vi "test.Cluster.vi"(8 "error in":errorcluster, 10 "Data":variant, 11 "Command":string) -> (0 "error out":errorcluster, 3 "Return Data":variant)   [LabVIEW 2014]
uses:
  Private/Class/class.GLue.lvclass
  Private/Class/meth.Constructor.vi
  Private/Class/meth.Destructor.vi
  GLue.lvlib
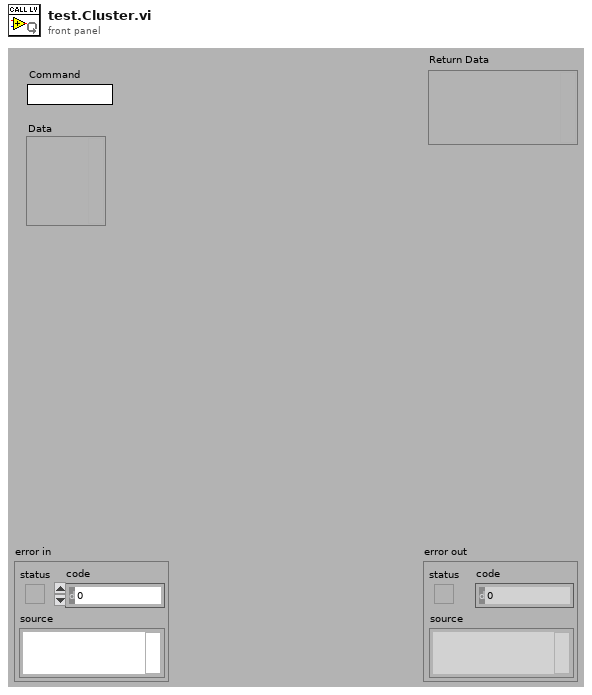
[diagram p1: front panel]
types:
  T1 = cluster{"bool":bool, "number":i32, "string":string, "ref":refnum<vi>}
  T2 = cluster{"ref":refnum<vi>, "df":string[][], "asd":cluster{"ref":refnum<vi>, "df":string[][]}[]}
  T3 = cluster{"arr":cluster{"ref":refnum<vi>, "df":string[][], "asd":cluster{"ref":refnum<vi>, "df":string[][]}[]}[]}
  T4 = cluster{"a":cluster{"bool":bool, "number":i32, "string":string}, "b":cluster{"bool":bool, "number":i32, "string":string, "c":cluster{"bool":bool, "number":i32, "string":string}}}
  T5 = cluster{"a":cluster{"bool":bool, "number":i32, "string":string}, "data":variant}
  T6 = cluster{"a":cluster{"numbers":i32[], "bools":bool[], "strings":string[]}, "b":cluster{"numbers":i32[], "bools":bool[], "strings":string[], "c":cluster{"numbers":i32[], "bools":bool[], "strings":string[]}}}
  T7 = cluster{"bool":bool, "number":i32, "string":string}
  T8 = cluster{"numbers":i32[], "bools":bool[], "strings":string[]}
  T9 = cluster{"numbers":i32[][], "bools":bool[][], "strings":string[][]}
  T10 = cluster{"ref":refnum<vi>, "df":string[][], "asd":cluster{"ref":refnum<vi>, "df":string[][]}[]}[]
  T11 = cluster{"a":refnum<vi>, "z":cluster{"array":string[][], "glue":refnum<class "class.GLue.lvclass">, "q":cluster{"a":refnum<vi>, "z":cluster{"array":string[][], "glue":refnum<class "class.GLue.lvclass">}[], "b":bool[], "c":refnum<queue>, "w":dbl[][], "d":cluster{"h":cluster{"i":picture, "j":variant, "g":path}, waveform(dbl)}}}[], "b":bool[], "c":refnum<queue>, "k 2":waveform(dbl), "d":cluster{"g":path, "h":cluster{"i":picture, "j":variant}}}
  T12 = cluster{"bool":bool, "number":i32, "string":string, "c":cluster{"bool":bool, "number":i32, "string":string}}
  T13 = cluster{"clus2":cluster{"clus1":cluster{bool, i32, "string":string}, string}, i32, "string":string}
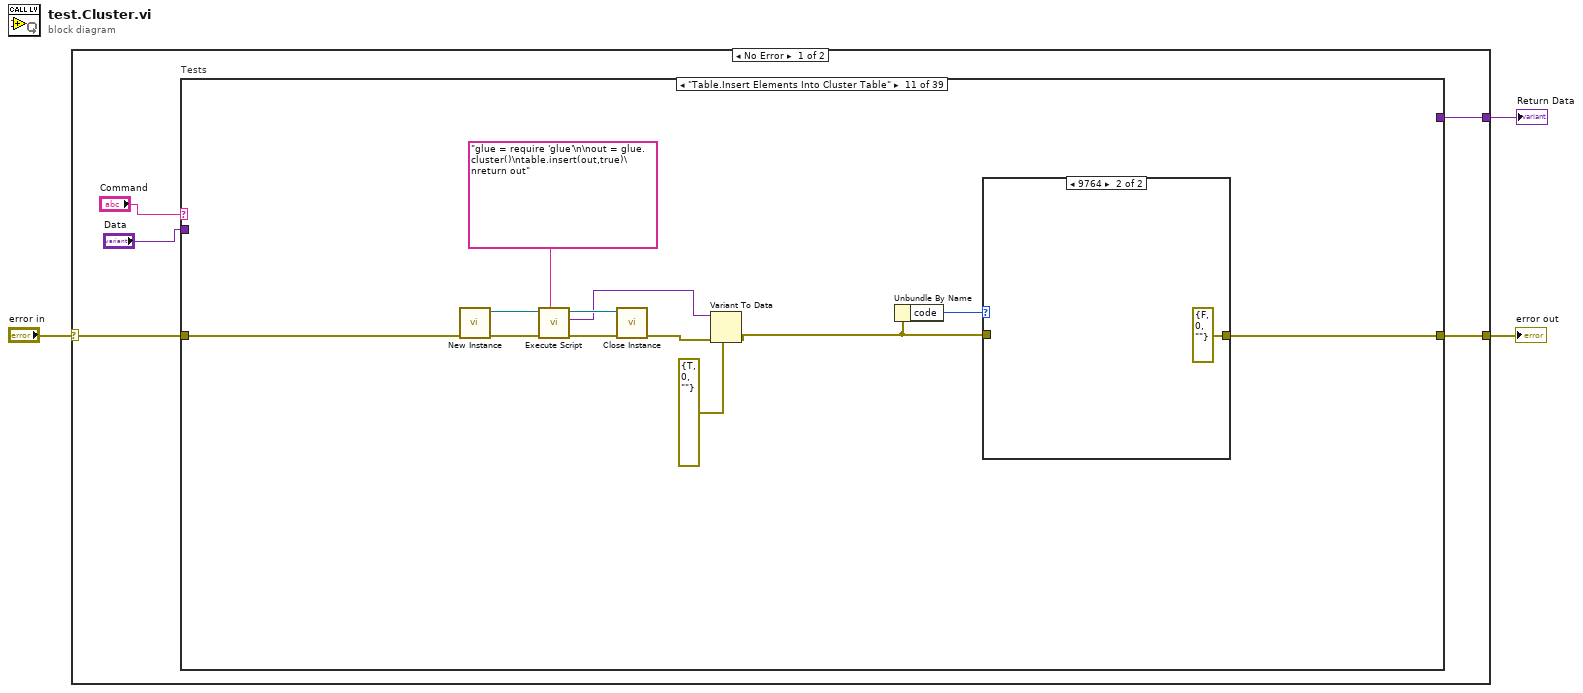
[diagram p0: block diagram]
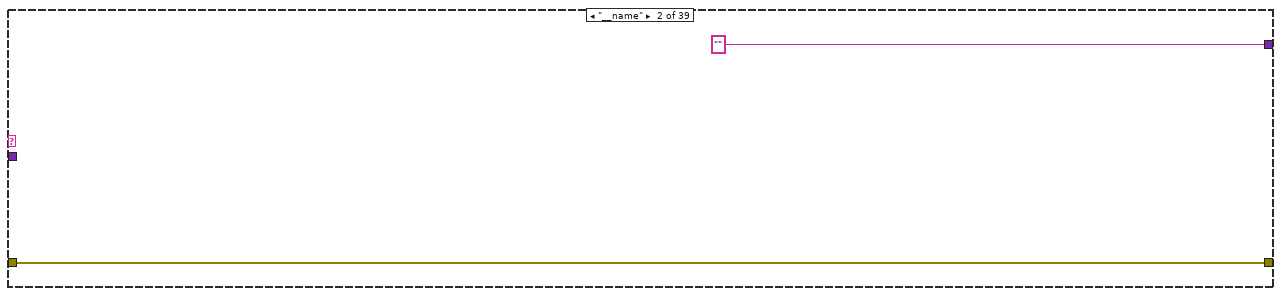
[diagram p3: hidden frame]
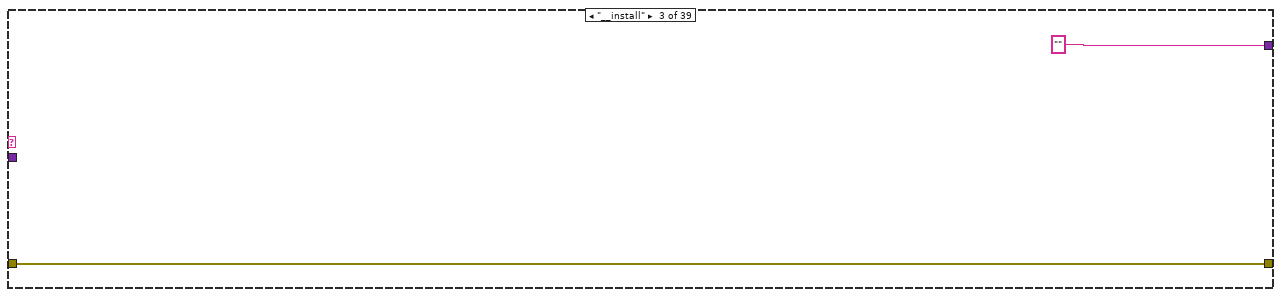
[diagram p4: hidden frame]
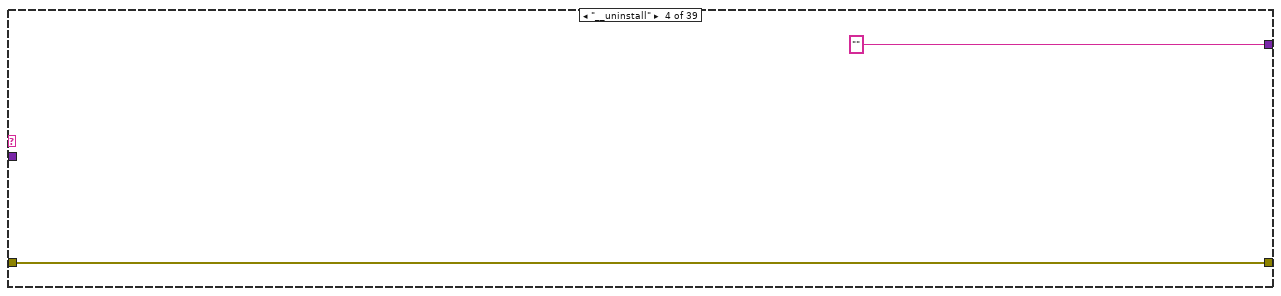
[diagram p5: hidden frame]
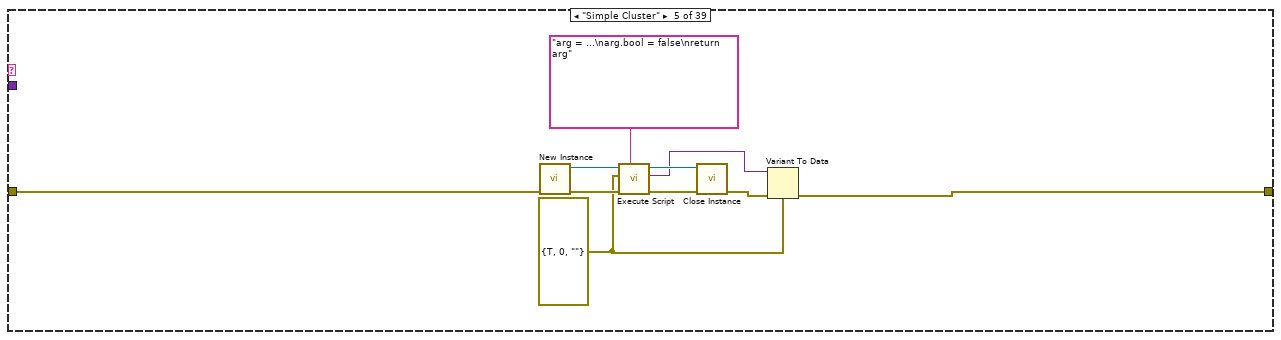
[diagram p6: hidden frame]
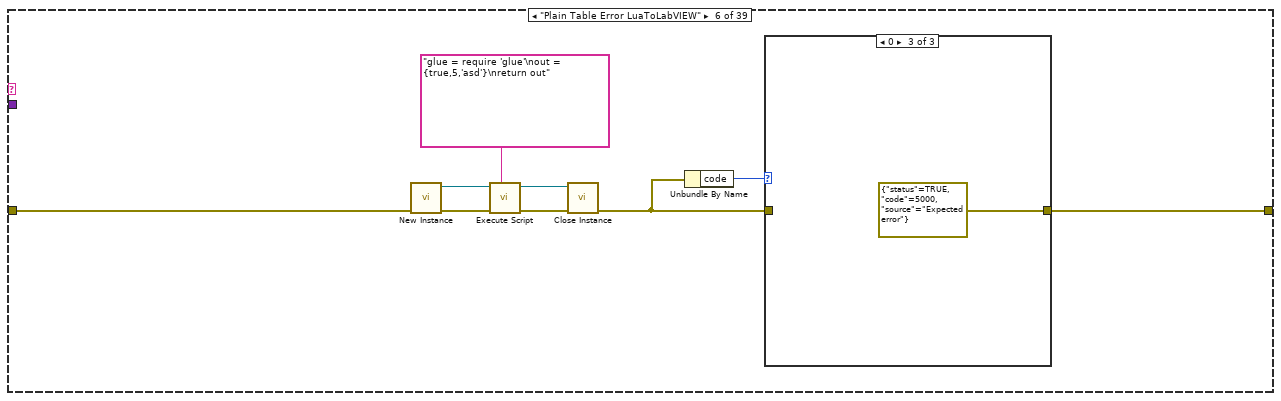
[diagram p7: hidden frame]
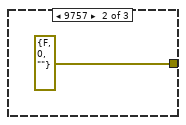
[diagram p9: hidden frame]
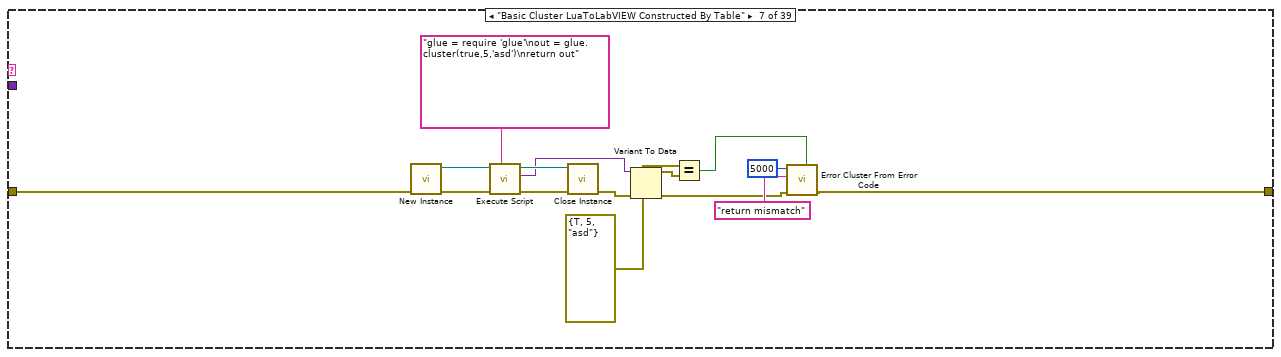
[diagram p10: hidden frame]
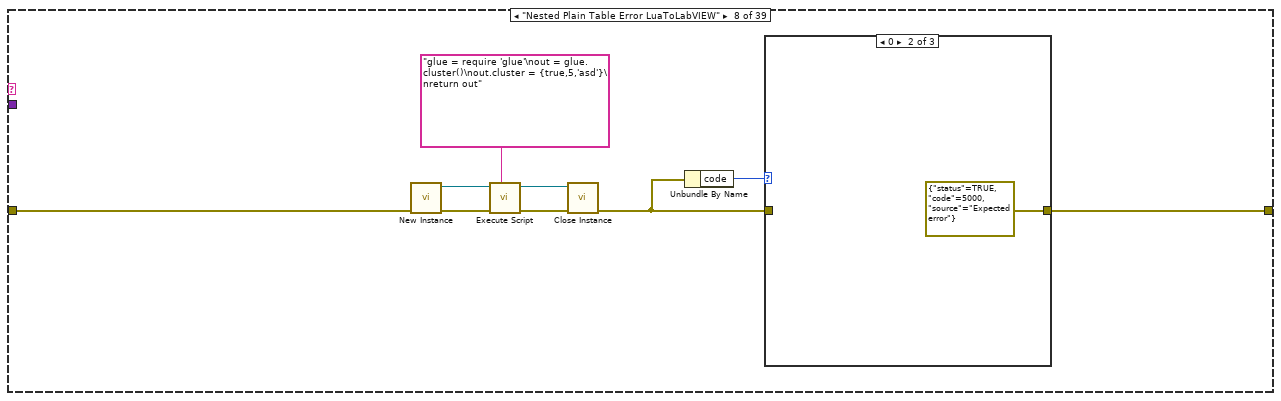
[diagram p11: hidden frame]
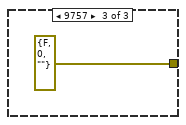
[diagram p13: hidden frame]
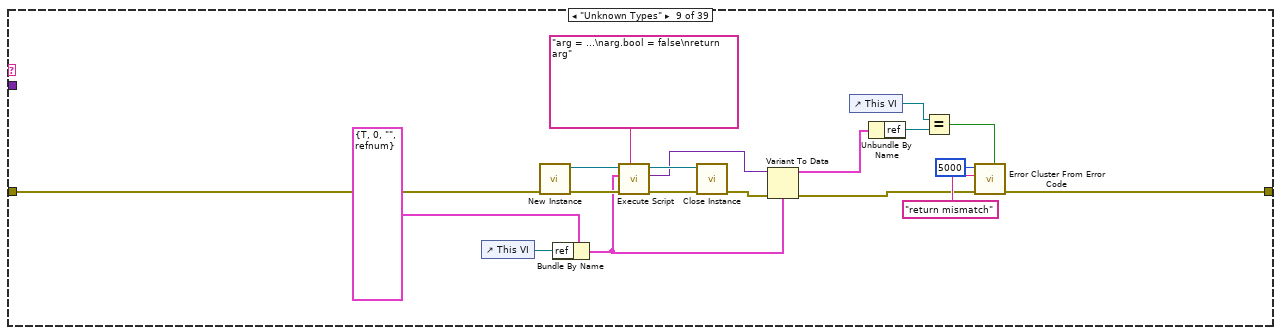
[diagram p14: hidden frame]
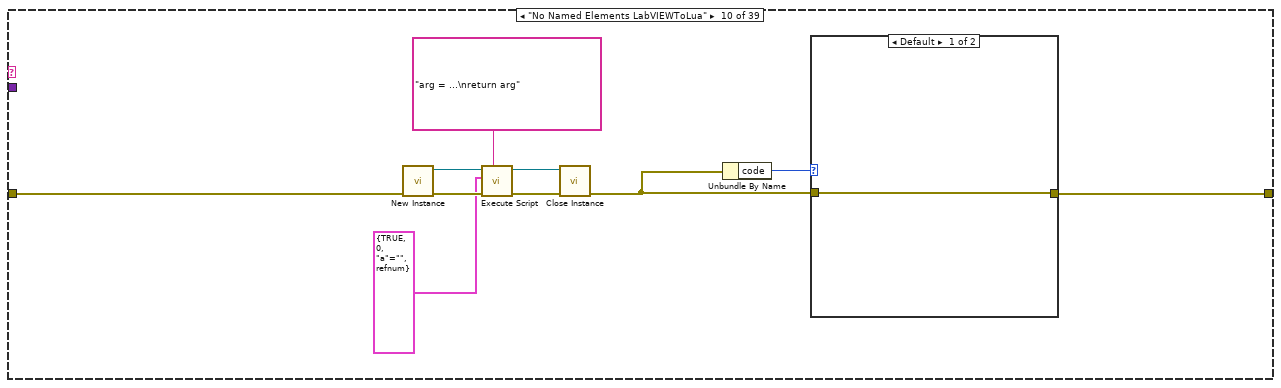
[diagram p15: hidden frame]
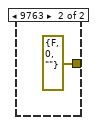
[diagram p16: hidden frame]
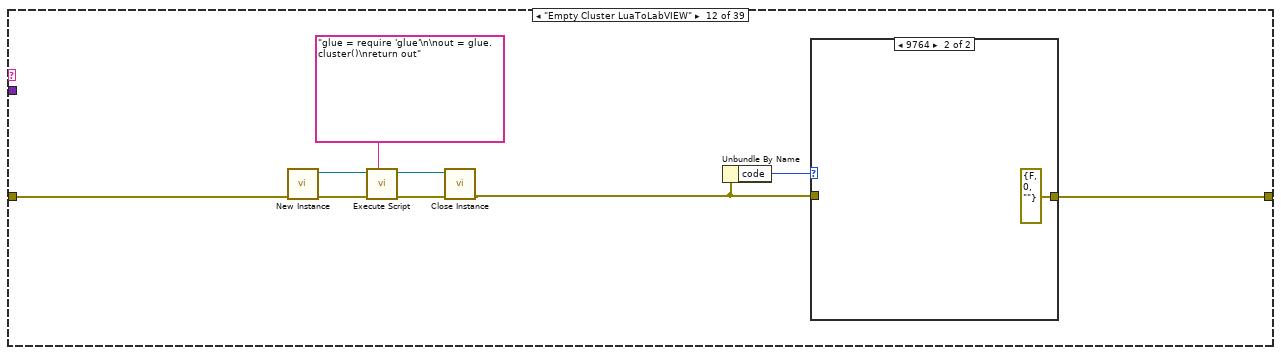
[diagram p18: hidden frame]
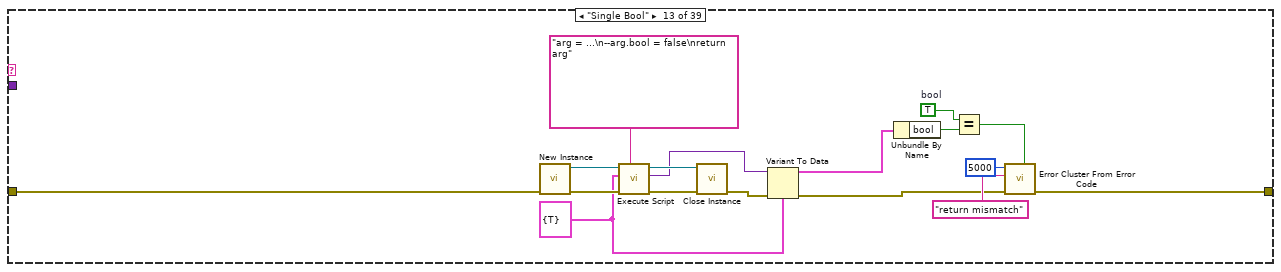
[diagram p20: hidden frame]
diagram:
  n1 = case shown="No Error" "error in" {
    selector: "error in" -> [w8 w594]
    tunnel: [w6 w594] -> w2
    tunnel: [w7 variant ("User Data")] -> w1
    frame No Error {
      n2 = case "Tests" shown="\"Table.Insert Elements Into Cluster Table\"" "Command" {
        tunnel: w8 -> [w10 w11 w13 w15 w21 w30 w48 w57 w79 w94 w108 w119 w133 w150 w167 w185 w204 w223 w253 w283 w305 w320 w335 w350 w365 w380 w395 w410 w425 w440 w458 w469 w496 w510 w526 w541 w557 w572 w580]
        tunnel: "Data" -> [w9 _ _ _ _ _ _ _ _ _ _ _ _ _ _ _ _ _ _ _ _ _ _ _ _ _ _ _ _ _ _ _ _ _ _ _ _ _ _]
        tunnel: [w9 "" "" "" _ _ _ _ _ _ _ _ _ _ _ _ _ _ _ _ _ _ _ _ _ _ _ _ _ _ _ _ _ _ _ _ _ _ _] -> w7
        tunnel: [w10 w11 w13 w15 w19 w28 w39 w55 w68 w93 w107 w118 w124 w142 w160 w180 w199 w218 w249 w279 w301 w316 w331 w346 w361 w376 w391 w406 w421 w436 w454 w465 w492 w509 w522 w532 w553 w568 w578] -> w6
        frame Default {
        }
        frame "__name" {
        }
        frame "__install" {
        }
        frame "__uninstall" {
        }
        frame "Simple Cluster" {
          w17 = T7 {"bool"=TRUE, "number"=0, "string"=""}
          n3 = call "New Instance.vi"("error in"=w21) -> ("error out"=w22:errorcluster, "GLue out"=w23:refnum<class "class.GLue.lvclass">)  [unwired: 9 in]
          n4 = call "Execute Script.vi"("Script"="arg = ...\narg.bool = false\nreturn arg", "error in"=w22, "Argument Data"=w17, "GLue in"=w23) -> ("error out"=w24:errorcluster, "Return Data"=w18:variant, "GLue out"=w25:refnum<class "class.GLue.lvclass">)  [unwired: 5 in]
          n5 = call "Close Instance.vi"("error in"=w24, "GLue in"=w25) -> ("error out"=w20:errorcluster)  [unwired: 9 in]
          n6 = Variant To Data(error in=w20, type=w17, Variant=w18) -> (error out=w19:errorcluster)  [unwired: 1 out]
        }
        frame "Plain Table Error LuaToLabVIEW" {
          n7 = call "New Instance.vi"("error in"=w30) -> ("error out"=w31:errorcluster, "GLue out"=w32:refnum<class "class.GLue.lvclass">)  [unwired: 9 in]
          n8 = call "Execute Script.vi"("Script"="glue = require 'glue'\nout = {true,5,'asd'}\nreturn out", "error in"=w31, "GLue in"=w32) -> ("error out"=w33:errorcluster, "GLue out"=w34:refnum<class "class.GLue.lvclass">)  [unwired: 6 in, 1 out]
          n9 = call "Close Instance.vi"("error in"=w33, "GLue in"=w34) -> ("error out"=w27:errorcluster)  [unwired: 9 in]
          n10 = Unbundle By Name(w27) -> ("code"=w29:i32)
          n11 = case shown="0" w29 {
            tunnel: [w36 errorcluster {"status"=FALSE, "code"=0, "source"=""} ("error out") errorcluster {"status"=TRUE, "code"=5000, "source"="Expected error"} ("error out")] -> w28
            tunnel: w27 -> [w36 _ _]
            frame Default {
            }
            frame 9757 {
            }
            frame 0 {
            }
          }
        }
        frame "Basic Cluster LuaToLabVIEW Constructed By Table" {
          w44 = T7 {"bool"=TRUE, "number"=5, "string"="asd"}
          n12 = call "New Instance.vi"("error in"=w48) -> ("error out"=w49:errorcluster, "GLue out"=w50:refnum<class "class.GLue.lvclass">)  [unwired: 9 in]
          n13 = call "Execute Script.vi"("Script"="glue = require 'glue'\nout = glue.cluster(true,5,'asd')\nreturn out", "error in"=w49, "GLue in"=w50) -> ("error out"=w51:errorcluster, "Return Data"=w46:variant, "GLue out"=w52:refnum<class "class.GLue.lvclass">)  [unwired: 6 in]
          n14 = call "Close Instance.vi"("error in"=w51, "GLue in"=w52) -> ("error out"=w47:errorcluster)  [unwired: 9 in]
          n15 = Variant To Data(error in=w47, type=w44, Variant=w46) -> (data=w45:T7, error out=w41:errorcluster)
          n16 = Equal?(x=w44, y=w45) -> (x = y?=w40:bool)
          n17 = call <vilib>:"Error Cluster From Error Code.vi"("is warning? (False)"=w40, "error in (no error)"=w41, "error message (\"\")"="return mismatch" ("error message (\"\")"), "error code (0)"=5000) -> ("error out"=w39:errorcluster)  [unwired: 5 in]
        }
        frame "Nested Plain Table Error LuaToLabVIEW" {
          n18 = call "New Instance.vi"("error in"=w57) -> ("error out"=w58:errorcluster, "GLue out"=w59:refnum<class "class.GLue.lvclass">)  [unwired: 9 in]
          n19 = call "Execute Script.vi"("Script"="glue = require 'glue'\nout = glue.cluster()\nout.cluster = {true,5,'asd'}\nreturn out", "error in"=w58, "GLue in"=w59) -> ("error out"=w60:errorcluster, "GLue out"=w61:refnum<class "class.GLue.lvclass">)  [unwired: 6 in, 1 out]
          n20 = call "Close Instance.vi"("error in"=w60, "GLue in"=w61) -> ("error out"=w54:errorcluster)  [unwired: 9 in]
          n21 = Unbundle By Name(w54) -> ("code"=w56:i32)
          n22 = case shown="0" w56 {
            tunnel: [w63 errorcluster {"status"=TRUE, "code"=5000, "source"="Expected error"} ("error out") errorcluster {"status"=FALSE, "code"=0, "source"=""} ("error out")] -> w55
            tunnel: w54 -> [w63 _ _]
            frame Default {
            }
            frame 0 {
            }
            frame 9757 {
            }
          }
        }
        frame "Unknown Types" {
          n23 = control-ref of="This VI"() -> (w74:refnum<vi>)
          n24 = call "New Instance.vi"("error in"=w79) -> ("error out"=w80:errorcluster, "GLue out"=w81:refnum<class "class.GLue.lvclass">)  [unwired: 9 in]
          n25 = Bundle By Name(cluster=T1 {"bool"=TRUE, "number"=0, "string"="", "ref"=refnum}, "ref"=w74) -> (w75:T1)
          n26 = call "Execute Script.vi"("Script"="arg = ...\narg.bool = false\nreturn arg", "error in"=w80, "Argument Data"=w75, "GLue in"=w81) -> ("error out"=w82:errorcluster, "Return Data"=w77:variant, "GLue out"=w83:refnum<class "class.GLue.lvclass">)  [unwired: 5 in]
          n27 = call "Close Instance.vi"("error in"=w82, "GLue in"=w83) -> ("error out"=w78:errorcluster)  [unwired: 9 in]
          n28 = Variant To Data(error in=w78, type=w75, Variant=w77) -> (data=w67:T1, error out=w69:errorcluster)
          n29 = control-ref of="This VI"() -> (w66:refnum<vi>)
          n30 = Unbundle By Name(w67) -> ("ref"=w73:refnum<vi>)
          n31 = Equal?(x=w66, y=w73) -> (x = y?=w72:bool)
          n32 = call <vilib>:"Error Cluster From Error Code.vi"("is warning? (False)"=w72, "error in (no error)"=w69, "error message (\"\")"="return mismatch" ("error message (\"\")"), "error code (0)"=5000) -> ("error out"=w68:errorcluster)  [unwired: 5 in]
        }
        frame "No Named Elements LabVIEWToLua" {
          n33 = call "New Instance.vi"("error in"=w94) -> ("error out"=w88:errorcluster, "GLue out"=w89:refnum<class "class.GLue.lvclass">)  [unwired: 9 in]
          n34 = call "Execute Script.vi"("Script"="arg = ...\nreturn arg", "error in"=w88, "Argument Data"=cluster{bool, i32, "a":string, refnum<vi>} {TRUE, 0, "a"="", refnum}, "GLue in"=w89) -> ("error out"=w90:errorcluster, "GLue out"=w91:refnum<class "class.GLue.lvclass">)  [unwired: 5 in, 1 out]
          n35 = call "Close Instance.vi"("error in"=w90, "GLue in"=w91) -> ("error out"=w85:errorcluster)  [unwired: 9 in]
          n36 = Unbundle By Name(w85) -> ("code"=w86:i32)
          n37 = case shown="Default" w86 {
            tunnel: [w95 errorcluster {"status"=FALSE, "code"=0, "source"=""} ("error out")] -> w93
            tunnel: w85 -> [w95 _]
            frame Default {
            }
            frame 9763 {
            }
          }
        }
        frame "Table.Insert Elements Into Cluster Table" {
          n38 = call "New Instance.vi"("error in"=w108) -> ("error out"=w102:errorcluster, "GLue out"=w103:refnum<class "class.GLue.lvclass">)  [unwired: 9 in]
          n39 = call "Execute Script.vi"("Script"="glue = require 'glue'\n\nout = glue.cluster()\ntable.insert(out,true)\nreturn out", "error in"=w102, "GLue in"=w103) -> ("error out"=w104:errorcluster, "Return Data"=w99:variant, "GLue out"=w105:refnum<class "class.GLue.lvclass">)  [unwired: 6 in]
          n40 = call "Close Instance.vi"("error in"=w104, "GLue in"=w105) -> ("error out"=w100:errorcluster)  [unwired: 9 in]
          n41 = Variant To Data(error in=w100, type=cluster{"a":bool, "b":i32, "c":string} {"a"=TRUE, "b"=0, "c"=""}, Variant=w99) -> (error out=w97:errorcluster)  [unwired: 1 out]
          n42 = Unbundle By Name(w97) -> ("code"=w101:i32)
          n43 = case shown="9764" w101 {
            tunnel: [w109 errorcluster {"status"=FALSE, "code"=0, "source"=""} ("error out")] -> w107
            tunnel: w97 -> [w109 _]
            frame Default {
            }
            frame 9764 {
            }
          }
        }
        frame "Empty Cluster LuaToLabVIEW" {
          n44 = call "New Instance.vi"("error in"=w119) -> ("error out"=w113:errorcluster, "GLue out"=w114:refnum<class "class.GLue.lvclass">)  [unwired: 9 in]
          n45 = call "Execute Script.vi"("Script"="glue = require 'glue'\n\nout = glue.cluster()\nreturn out", "error in"=w113, "GLue in"=w114) -> ("error out"=w115:errorcluster, "GLue out"=w116:refnum<class "class.GLue.lvclass">)  [unwired: 6 in, 1 out]
          n46 = call "Close Instance.vi"("error in"=w115, "GLue in"=w116) -> ("error out"=w111:errorcluster)  [unwired: 9 in]
          n47 = Unbundle By Name(w111) -> ("code"=w112:i32)
          n48 = case shown="9764" w112 {
            tunnel: [w120 errorcluster {"status"=FALSE, "code"=0, "source"=""} ("error out")] -> w118
            tunnel: w111 -> [w120 _]
            frame Default {
            }
            frame 9764 {
            }
          }
        }
        frame "Single Bool" {
          w122 = TRUE  # bool
          w130 = cluster{"bool":bool} {"bool"=TRUE}
          n49 = call "New Instance.vi"("error in"=w133) -> ("error out"=w134:errorcluster, "GLue out"=w135:refnum<class "class.GLue.lvclass">)  [unwired: 9 in]
          n50 = call "Execute Script.vi"("Script"="arg = ...\n--arg.bool = false\nreturn arg", "error in"=w134, "Argument Data"=w130, "GLue in"=w135) -> ("error out"=w136:errorcluster, "Return Data"=w131:variant, "GLue out"=w137:refnum<class "class.GLue.lvclass">)  [unwired: 5 in]
          n51 = call "Close Instance.vi"("error in"=w136, "GLue in"=w137) -> ("error out"=w132:errorcluster)  [unwired: 9 in]
          n52 = Variant To Data(error in=w132, type=w130, Variant=w131) -> (data=w123:cluster{"bool":bool}, error out=w125:errorcluster)
          n53 = Unbundle By Name(w123) -> ("bool"=w129:bool)
          n54 = Equal?(x=w122, y=w129) -> (x = y?=w128:bool)
          n55 = call <vilib>:"Error Cluster From Error Code.vi"("is warning? (False)"=w128, "error in (no error)"=w125, "error message (\"\")"="return mismatch" ("error message (\"\")"), "error code (0)"=5000) -> ("error out"=w124:errorcluster)  [unwired: 5 in]
        }
        frame "Single Number" {
          w147 = cluster{"number":dbl} {"number"=0.0}
          n56 = call "New Instance.vi"("error in"=w150) -> ("error out"=w151:errorcluster, "GLue out"=w152:refnum<class "class.GLue.lvclass">)  [unwired: 9 in]
          n57 = call "Execute Script.vi"("Script"="arg = ...\narg.number = 10\nreturn arg", "error in"=w151, "Argument Data"=w147, "GLue in"=w152) -> ("error out"=w153:errorcluster, "Return Data"=w148:variant, "GLue out"=w154:refnum<class "class.GLue.lvclass">)  [unwired: 5 in]
          n58 = call "Close Instance.vi"("error in"=w153, "GLue in"=w154) -> ("error out"=w149:errorcluster)  [unwired: 9 in]
          n59 = Variant To Data(error in=w149, type=w147, Variant=w148) -> (data=w146:cluster{"number":dbl}, error out=w143:errorcluster)
          n60 = Unbundle By Name(w146) -> ("number"=w145:dbl)
          n61 = Equal?(x=10.0, y=w145) -> (x = y?=w141:bool)
          n62 = call <vilib>:"Error Cluster From Error Code.vi"("is warning? (False)"=w141, "error in (no error)"=w143, "error message (\"\")"="return mismatch" ("error message (\"\")"), "error code (0)"=5000) -> ("error out"=w142:errorcluster)  [unwired: 5 in]
        }
        frame "Single String" {
          w164 = cluster{"string":string} {"string"="hallo"}
          n63 = call "New Instance.vi"("error in"=w167) -> ("error out"=w168:errorcluster, "GLue out"=w169:refnum<class "class.GLue.lvclass">)  [unwired: 9 in]
          n64 = call "Execute Script.vi"("Script"="arg = ...\narg.string = 'foo'\nreturn arg", "error in"=w168, "Argument Data"=w164, "GLue in"=w169) -> ("error out"=w170:errorcluster, "Return Data"=w165:variant, "GLue out"=w171:refnum<class "class.GLue.lvclass">)  [unwired: 5 in]
          n65 = call "Close Instance.vi"("error in"=w170, "GLue in"=w171) -> ("error out"=w166:errorcluster)  [unwired: 9 in]
          n66 = Variant To Data(error in=w166, type=w164, Variant=w165) -> (data=w163:cluster{"string":string}, error out=w161:errorcluster)
          n67 = Unbundle By Name(w163) -> ("string"=w162:string)
          n68 = Equal?(x="foo" ("error message (\"\")"), y=w162) -> (x = y?=w159:bool)
          n69 = call <vilib>:"Error Cluster From Error Code.vi"("is warning? (False)"=w159, "error in (no error)"=w161, "error message (\"\")"="return mismatch" ("error message (\"\")"), "error code (0)"=5000) -> ("error out"=w160:errorcluster)  [unwired: 5 in]
        }
        frame "1dString Array" {
          w177 = cluster{"array":string[]} {"array"=["a", "b", "c"]}
          n70 = call "New Instance.vi"("error in"=w185) -> ("error out"=w186:errorcluster, "GLue out"=w187:refnum<class "class.GLue.lvclass">)  [unwired: 9 in]
          n71 = call "Execute Script.vi"("Script"="arg = ...\narg.array[1] = 'foo'\nreturn arg", "error in"=w186, "Argument Data"=w177, "GLue in"=w187) -> ("error out"=w188:errorcluster, "Return Data"=w183:variant, "GLue out"=w189:refnum<class "class.GLue.lvclass">)  [unwired: 5 in]
          n72 = call "Close Instance.vi"("error in"=w188, "GLue in"=w189) -> ("error out"=w184:errorcluster)  [unwired: 9 in]
          n73 = Variant To Data(error in=w184, type=w177, Variant=w183) -> (data=w182:cluster{"array":string[]}, error out=w181:errorcluster)
          n74 = Unbundle By Name(w182) -> ("array"=w176:string[])
          n75 = Index Array(array=w176) -> (element=w175:string)  [unwired: 1 in]
          n76 = Equal?(x=w175, y="foo" ("error message (\"\")")) -> (x = y?=w173:bool)
          n77 = call <vilib>:"Error Cluster From Error Code.vi"("is warning? (False)"=w173, "error in (no error)"=w181, "error message (\"\")"="return mismatch" ("error message (\"\")"), "error code (0)"=5000) -> ("error out"=w180:errorcluster)  [unwired: 5 in]
        }
        frame "1dBool Array" {
          w196 = cluster{"array":bool[]} {"array"=[FALSE, FALSE, FALSE]}
          n78 = call "New Instance.vi"("error in"=w204) -> ("error out"=w205:errorcluster, "GLue out"=w206:refnum<class "class.GLue.lvclass">)  [unwired: 9 in]
          n79 = call "Execute Script.vi"("Script"="arg = ...\narg.array[2] = true\nreturn arg", "error in"=w205, "Argument Data"=w196, "GLue in"=w206) -> ("error out"=w207:errorcluster, "Return Data"=w202:variant, "GLue out"=w208:refnum<class "class.GLue.lvclass">)  [unwired: 5 in]
          n80 = call "Close Instance.vi"("error in"=w207, "GLue in"=w208) -> ("error out"=w203:errorcluster)  [unwired: 9 in]
          n81 = Variant To Data(error in=w203, type=w196, Variant=w202) -> (data=w201:cluster{"array":bool[]}, error out=w200:errorcluster)
          n82 = Unbundle By Name(w201) -> ("array"=w195:bool[])
          n83 = Index Array(array=w195, index=1) -> (element=w194:bool)
          n84 = Equal?(x=w194, y=TRUE ("element")) -> (x = y?=w193:bool)
          n85 = call <vilib>:"Error Cluster From Error Code.vi"("is warning? (False)"=w193, "error in (no error)"=w200, "error message (\"\")"="return mismatch" ("error message (\"\")"), "error code (0)"=5000) -> ("error out"=w199:errorcluster)  [unwired: 5 in]
        }
        frame "1dNumber Array" {
          w215 = cluster{"array":i32[]} {"array"=[1, 2, 3]}
          n86 = call "New Instance.vi"("error in"=w223) -> ("error out"=w224:errorcluster, "GLue out"=w225:refnum<class "class.GLue.lvclass">)  [unwired: 9 in]
          n87 = call "Execute Script.vi"("Script"="arg = ...\narg.array[2] = 5\nreturn arg", "error in"=w224, "Argument Data"=w215, "GLue in"=w225) -> ("error out"=w226:errorcluster, "Return Data"=w221:variant, "GLue out"=w227:refnum<class "class.GLue.lvclass">)  [unwired: 5 in]
          n88 = call "Close Instance.vi"("error in"=w226, "GLue in"=w227) -> ("error out"=w222:errorcluster)  [unwired: 9 in]
          n89 = Variant To Data(error in=w222, type=w215, Variant=w221) -> (data=w220:cluster{"array":i32[]}, error out=w219:errorcluster)
          n90 = Unbundle By Name(w220) -> ("array"=w214:i32[])
          n91 = Index Array(array=w214, index=1) -> (element=w213:i32)
          n92 = Equal?(x=w213, y=5 ("index")) -> (x = y?=w212:bool)
          n93 = call <vilib>:"Error Cluster From Error Code.vi"("is warning? (False)"=w212, "error in (no error)"=w219, "error message (\"\")"="return mismatch" ("error message (\"\")"), "error code (0)"=5000) -> ("error out"=w218:errorcluster)  [unwired: 5 in]
        }
        frame "Basic Arrays" {
          w246 = T8 {"numbers"=[1, 2, 3], "bools"=[FALSE, FALSE, FALSE], "strings"=["a", "b", "c"]}
          n94 = call "New Instance.vi"("error in"=w253) -> ("error out"=w254:errorcluster, "GLue out"=w255:refnum<class "class.GLue.lvclass">)  [unwired: 9 in]
          n95 = call "Execute Script.vi"("Script"="arg = ...\narg.numbers[2] = 5\narg.bools[2] = true\narg.strings[2] = 'g'\nreturn arg", "error in"=w254, "Argument Data"=w246, "GLue in"=w255) -> ("error out"=w256:errorcluster, "Return Data"=w251:variant, "GLue out"=w257:refnum<class "class.GLue.lvclass">)  [unwired: 5 in]
          n96 = call "Close Instance.vi"("error in"=w256, "GLue in"=w257) -> ("error out"=w252:errorcluster)  [unwired: 9 in]
          n97 = Variant To Data(error in=w252, type=w246, Variant=w251) -> (data=w234:T8, error out=w250:errorcluster)
          n98 = Unbundle By Name(w234) -> ("strings"=w237:string[])
          n99 = Unbundle By Name(w234) -> ("numbers"=w245:i32[])
          n100 = Unbundle By Name(w234) -> ("bools"=w239:bool[])
          n101 = Index Array(array=w237, index=1) -> (element=w236:string)
          n102 = Index Array(array=w239, index=1) -> (element=w240:bool)
          n103 = Index Array(array=w245, index=1) -> (element=w244:i32)
          n104 = Equal?(x=w236, y="g") -> (x = y?=w230:bool)
          n105 = Equal?(x=w240, y=TRUE) -> (x = y?=w231:bool)
          n106 = Equal?(x=w244, y=5 ("index")) -> (x = y?=w232:bool)
          n107 = Compound Arithmetic op=AND(w232, w231, w230) -> (w229:bool)
          n108 = call <vilib>:"Error Cluster From Error Code.vi"("is warning? (False)"=w229, "error in (no error)"=w250, "error message (\"\")"="return mismatch" ("error message (\"\")"), "error code (0)"=5000) -> ("error out"=w249:errorcluster)  [unwired: 5 in]
        }
        frame "Basic 2d Arrays" {
          w259 = 1 ("index")
          w261 = 1 ("index")
          w260 = 1 ("index")
          w276 = T9 {"numbers"=[[1, 2, 3], [3, 4, 0]], "bools"=[[FALSE, FALSE, FALSE], [TRUE, TRUE, TRUE]], "strings"=[["a", "b", "c"], ["c", "d", "hallo"]]}
          n109 = call "New Instance.vi"("error in"=w283) -> ("error out"=w284:errorcluster, "GLue out"=w285:refnum<class "class.GLue.lvclass">)  [unwired: 9 in]
          n110 = call "Execute Script.vi"("Script"="arg = ...\narg.numbers[2][2] = 5\narg.bools[2][2] = true\narg.strings[2][2] = 'g'\nreturn arg", "error in"=w284, "Argument Data"=w276, "GLue in"=w285) -> ("error out"=w286:errorcluster, "Return Data"=w281:variant, "GLue out"=w287:refnum<class "class.GLue.lvclass">)  [unwired: 5 in]
          n111 = call "Close Instance.vi"("error in"=w286, "GLue in"=w287) -> ("error out"=w282:errorcluster)  [unwired: 9 in]
          n112 = Variant To Data(error in=w282, type=w276, Variant=w281) -> (data=w267:T9, error out=w280:errorcluster)
          n113 = Unbundle By Name(w267) -> ("strings"=w269:string[][])
          n114 = Unbundle By Name(w267) -> ("numbers"=w275:i32[][])
          n115 = Unbundle By Name(w267) -> ("bools"=w271:bool[][])
          n116 = Index Array(array=w269, index (row)=w259, index (col)=w259) -> (element=w268:string)
          n117 = Index Array(array=w271, index (row)=w261, index (col)=w261) -> (element=w272:bool)
          n118 = Index Array(array=w275, index (row)=w260, index (col)=w260) -> (element=w274:i32)
          n119 = Equal?(x=w268, y="g") -> (x = y?=w263:bool)
          n120 = Equal?(x=w272, y=TRUE) -> (x = y?=w264:bool)
          n121 = Equal?(x=w274, y=5 ("index")) -> (x = y?=w265:bool)
          n122 = Compound Arithmetic op=AND(w265, w264, w263) -> (w262:bool)
          n123 = call <vilib>:"Error Cluster From Error Code.vi"("is warning? (False)"=w262, "error in (no error)"=w280, "error message (\"\")"="return mismatch" ("error message (\"\")"), "error code (0)"=5000) -> ("error out"=w279:errorcluster)  [unwired: 5 in]
        }
        frame "Nested Cluster Array" {
          n124 = control-ref of="This VI"() -> (w297:refnum<vi>)
          n125 = Bundle By Name(cluster=cluster{"ref":refnum<vi>} {"ref"=refnum}, "ref"=w297) -> (w294:cluster{"ref":refnum<vi>})
          n126 = Build Array(w294, w294, w294, w294) -> (w293:cluster{"ref":refnum<vi>}[])
          n127 = call "New Instance.vi"("error in"=w305) -> ("error out"=w306:errorcluster, "GLue out"=w307:refnum<class "class.GLue.lvclass">)  [unwired: 9 in]
          n128 = Bundle By Name(cluster=cluster{"arr":cluster{"ref":refnum<vi>}[]} {"arr"=[]}, "arr"=w293) -> (w295:cluster{"arr":cluster{"ref":refnum<vi>}[]})
          n129 = call "Execute Script.vi"("Script"="arg = ...\nreturn arg.arr[3].ref", "error in"=w306, "Argument Data"=w295, "GLue in"=w307) -> ("error out"=w308:errorcluster, "Return Data"=w303:variant, "GLue out"=w309:refnum<class "class.GLue.lvclass">)  [unwired: 5 in]
          n130 = call "Close Instance.vi"("error in"=w308, "GLue in"=w309) -> ("error out"=w304:errorcluster)  [unwired: 9 in]
          n131 = Variant To Data(error in=w304, type=refnum<vi> refnum ("ref"), Variant=w303) -> (data=w290:refnum<vi>, error out=w302:errorcluster)
          n132 = control-ref of="This VI"() -> (w291:refnum<vi>)
          n133 = Equal?(x=w291, y=w290) -> (x = y?=w289:bool)
          n134 = call <vilib>:"Error Cluster From Error Code.vi"("is warning? (False)"=w289, "error in (no error)"=w302, "error message (\"\")"="return mismatch" ("error message (\"\")"), "error code (0)"=5000) -> ("error out"=w301:errorcluster)  [unwired: 5 in]
        }
        frame "Cluster Array LuaToLabVIEW Embedded Strings" {
          w311 = cluster{string}[] [{"asd"}, {"qwe"}, {"zxc"}]
          n135 = call "New Instance.vi"("error in"=w320) -> ("error out"=w321:errorcluster, "GLue out"=w322:refnum<class "class.GLue.lvclass">)  [unwired: 9 in]
          n136 = call "Execute Script.vi"("Script"="g = require 'glue'\nout = g.clusterArray()\nout[1] = g.cluster('asd')\nout[2] = g.cluster('qwe')\nout[3] = g.cluster('zxc')\nreturn out", "error in"=w321, "GLue in"=w322) -> ("error out"=w323:errorcluster, "Return Data"=w318:variant, "GLue out"=w324:refnum<class "class.GLue.lvclass">)  [unwired: 6 in]
          n137 = call "Close Instance.vi"("error in"=w323, "GLue in"=w324) -> ("error out"=w319:errorcluster)  [unwired: 9 in]
          n138 = Variant To Data(error in=w319, type=w311, Variant=w318) -> (data=w312:cluster{string}[], error out=w317:errorcluster)
          n139 = Equal?(x=w312, y=w311) -> (x = y?=w313:bool)
          n140 = call <vilib>:"Error Cluster From Error Code.vi"("is warning? (False)"=w313, "error in (no error)"=w317, "error message (\"\")"="return mismatch" ("error message (\"\")"), "error code (0)"=5000) -> ("error out"=w316:errorcluster)  [unwired: 5 in]
        }
        frame "Cluster Array LuaToLabVIEW Embedded Numbers" {
          w326 = cluster{dbl}[] [{5.0}, {6.0}, {7.0}]
          n141 = call "New Instance.vi"("error in"=w335) -> ("error out"=w336:errorcluster, "GLue out"=w337:refnum<class "class.GLue.lvclass">)  [unwired: 9 in]
          n142 = call "Execute Script.vi"("Script"="g = require 'glue'\nout = g.clusterArray()\nout[1] = g.cluster(5)\nout[2] = g.cluster(6)\nout[3] = g.cluster(7)\nreturn out", "error in"=w336, "GLue in"=w337) -> ("error out"=w338:errorcluster, "Return Data"=w333:variant, "GLue out"=w339:refnum<class "class.GLue.lvclass">)  [unwired: 6 in]
          n143 = call "Close Instance.vi"("error in"=w338, "GLue in"=w339) -> ("error out"=w334:errorcluster)  [unwired: 9 in]
          n144 = Variant To Data(error in=w334, type=w326, Variant=w333) -> (data=w327:cluster{dbl}[], error out=w332:errorcluster)
          n145 = Equal?(x=w327, y=w326) -> (x = y?=w328:bool)
          n146 = call <vilib>:"Error Cluster From Error Code.vi"("is warning? (False)"=w328, "error in (no error)"=w332, "error message (\"\")"="return mismatch" ("error message (\"\")"), "error code (0)"=5000) -> ("error out"=w331:errorcluster)  [unwired: 5 in]
        }
        frame "Cluster Array LuaToLabVIEW Embedded Bools" {
          w341 = cluster{bool}[] [{TRUE}, {FALSE}, {TRUE}]
          n147 = call "New Instance.vi"("error in"=w350) -> ("error out"=w351:errorcluster, "GLue out"=w352:refnum<class "class.GLue.lvclass">)  [unwired: 9 in]
          n148 = call "Execute Script.vi"("Script"="g = require 'glue'\nout = g.clusterArray()\nout[1] = g.cluster(true)\nout[2] = g.cluster(false)\nout[3] = g.cluster(true)\nreturn out", "error in"=w351, "GLue in"=w352) -> ("error out"=w353:errorcluster, "Return Data"=w348:variant, "GLue out"=w354:refnum<class "class.GLue.lvclass">)  [unwired: 6 in]
          n149 = call "Close Instance.vi"("error in"=w353, "GLue in"=w354) -> ("error out"=w349:errorcluster)  [unwired: 9 in]
          n150 = Variant To Data(error in=w349, type=w341, Variant=w348) -> (data=w342:cluster{bool}[], error out=w347:errorcluster)
          n151 = Equal?(x=w342, y=w341) -> (x = y?=w343:bool)
          n152 = call <vilib>:"Error Cluster From Error Code.vi"("is warning? (False)"=w343, "error in (no error)"=w347, "error message (\"\")"="return mismatch" ("error message (\"\")"), "error code (0)"=5000) -> ("error out"=w346:errorcluster)  [unwired: 5 in]
        }
        frame "Cluster Array LuaToLabVIEW Embedded String Array" {
          w356 = cluster{string[]}[] [{["a", "s", "d"]}, {["q", "w", "e"]}, {["z", "x", "c"]}]
          n153 = call "New Instance.vi"("error in"=w365) -> ("error out"=w366:errorcluster, "GLue out"=w367:refnum<class "class.GLue.lvclass">)  [unwired: 9 in]
          n154 = call "Execute Script.vi"("Script"="g = require 'glue'\nout = g.clusterArray()\nout[1] = g.cluster(g.stringArray('a','s','d'))\nout[2] = g.cluster(g.stringArray('q','w','e'))\nout[3] = g.cluster(g.stringArray('z','x','c'))\nreturn out", "error in"=w366, "GLue in"=w367) -> ("error out"=w368:errorcluster, "Return Data"=w363:variant, "GLue out"=w369:refnum<class "class.GLue.lvclass">)  [unwired: 6 in]
          n155 = call "Close Instance.vi"("error in"=w368, "GLue in"=w369) -> ("error out"=w364:errorcluster)  [unwired: 9 in]
          n156 = Variant To Data(error in=w364, type=w356, Variant=w363) -> (data=w357:cluster{string[]}[], error out=w362:errorcluster)
          n157 = Equal?(x=w357, y=w356) -> (x = y?=w358:bool)
          n158 = call <vilib>:"Error Cluster From Error Code.vi"("is warning? (False)"=w358, "error in (no error)"=w362, "error message (\"\")"="return mismatch" ("error message (\"\")"), "error code (0)"=5000) -> ("error out"=w361:errorcluster)  [unwired: 5 in]
        }
        frame "Cluster Array LuaToLabVIEW Embedded Bool Array" {
          w371 = cluster{bool[]}[] [{[FALSE, TRUE, FALSE]}, {[TRUE, FALSE, TRUE]}, {[FALSE, TRUE, FALSE]}]
          n159 = call "New Instance.vi"("error in"=w380) -> ("error out"=w381:errorcluster, "GLue out"=w382:refnum<class "class.GLue.lvclass">)  [unwired: 9 in]
          n160 = call "Execute Script.vi"("Script"="g = require 'glue'\nout = g.clusterArray()\nout[1] = g.cluster(g.boolArray(false,true,false))\nout[2] = g.cluster(g.boolArray(true,false,true))\nout[3] = g.cluster(g.boolArray(false,true,false))\nreturn out", "error in"=w381, "GLue in"=w382) -> ("error out"=w383:errorcluster, "Return Data"=w378:variant, "GLue out"=w384:refnum<class "class.GLue.lvclass">)  [unwired: 6 in]
          n161 = call "Close Instance.vi"("error in"=w383, "GLue in"=w384) -> ("error out"=w379:errorcluster)  [unwired: 9 in]
          n162 = Variant To Data(error in=w379, type=w371, Variant=w378) -> (data=w372:cluster{bool[]}[], error out=w377:errorcluster)
          n163 = Equal?(x=w372, y=w371) -> (x = y?=w373:bool)
          n164 = call <vilib>:"Error Cluster From Error Code.vi"("is warning? (False)"=w373, "error in (no error)"=w377, "error message (\"\")"="return mismatch" ("error message (\"\")"), "error code (0)"=5000) -> ("error out"=w376:errorcluster)  [unwired: 5 in]
        }
        frame "Cluster Array LuaToLabVIEW Embedded Bool Array Jagged" {
          w386 = cluster{bool[]}[] [{[FALSE, TRUE, FALSE]}, {[]}, {[FALSE, TRUE, FALSE]}]
          n165 = call "New Instance.vi"("error in"=w395) -> ("error out"=w396:errorcluster, "GLue out"=w397:refnum<class "class.GLue.lvclass">)  [unwired: 9 in]
          n166 = call "Execute Script.vi"("Script"="g = require 'glue'\nout = g.clusterArray()\nout[1] = g.cluster(g.boolArray(false,true,false))\nout[2] = g.cluster(g.boolArray())\nout[3] = g.cluster(g.boolArray(false,true,false))\nreturn out", "error in"=w396, "GLue in"=w397) -> ("error out"=w398:errorcluster, "Return Data"=w393:variant, "GLue out"=w399:refnum<class "class.GLue.lvclass">)  [unwired: 6 in]
          n167 = call "Close Instance.vi"("error in"=w398, "GLue in"=w399) -> ("error out"=w394:errorcluster)  [unwired: 9 in]
          n168 = Variant To Data(error in=w394, type=w386, Variant=w393) -> (data=w387:cluster{bool[]}[], error out=w392:errorcluster)
          n169 = Equal?(x=w387, y=w386) -> (x = y?=w388:bool)
          n170 = call <vilib>:"Error Cluster From Error Code.vi"("is warning? (False)"=w388, "error in (no error)"=w392, "error message (\"\")"="return mismatch" ("error message (\"\")"), "error code (0)"=5000) -> ("error out"=w391:errorcluster)  [unwired: 5 in]
        }
        frame "Cluster Array LuaToLabVIEW Embedded Bool Array Constructed" {
          w401 = cluster{bool[]}[] [{[FALSE, TRUE, FALSE]}, {[TRUE, FALSE, TRUE]}, {[FALSE, TRUE, FALSE]}]
          n171 = call "New Instance.vi"("error in"=w410) -> ("error out"=w411:errorcluster, "GLue out"=w412:refnum<class "class.GLue.lvclass">)  [unwired: 9 in]
          n172 = call "Execute Script.vi"("Script"="g = require 'glue'\nout = g.clusterArray(g.cluster(g.boolArray(false,true,false)),g.cluster(g.boolArray(true,false,true)),g.cluster(g.boolArray(false,true,false)))\nreturn out", "error in"=w411, "GLue in"=w412) -> ("error out"=w413:errorcluster, "Return Data"=w408:variant, "GLue out"=w414:refnum<class "class.GLue.lvclass">)  [unwired: 6 in]
          n173 = call "Close Instance.vi"("error in"=w413, "GLue in"=w414) -> ("error out"=w409:errorcluster)  [unwired: 9 in]
          n174 = Variant To Data(error in=w409, type=w401, Variant=w408) -> (data=w402:cluster{bool[]}[], error out=w407:errorcluster)
          n175 = Equal?(x=w402, y=w401) -> (x = y?=w403:bool)
          n176 = call <vilib>:"Error Cluster From Error Code.vi"("is warning? (False)"=w403, "error in (no error)"=w407, "error message (\"\")"="return mismatch" ("error message (\"\")"), "error code (0)"=5000) -> ("error out"=w406:errorcluster)  [unwired: 5 in]
        }
        frame "Cluster Array LuaToLabVIEW Embedded String Array Constructed" {
          w416 = cluster{string[]}[] [{["a", "s", "d"]}, {["q", "w", "e"]}, {["z", "x", "c"]}]
          n177 = call "New Instance.vi"("error in"=w425) -> ("error out"=w426:errorcluster, "GLue out"=w427:refnum<class "class.GLue.lvclass">)  [unwired: 9 in]
          n178 = call "Execute Script.vi"("Script"="g = require 'glue'\nout = g.clusterArray(g.cluster(g.stringArray('a','s','d')),g.cluster(g.stringArray('q','w','e')),g.cluster(g.stringArray('z','x','c')))\nreturn out", "error in"=w426, "GLue in"=w427) -> ("error out"=w428:errorcluster, "Return Data"=w423:variant, "GLue out"=w429:refnum<class "class.GLue.lvclass">)  [unwired: 6 in]
          n179 = call "Close Instance.vi"("error in"=w428, "GLue in"=w429) -> ("error out"=w424:errorcluster)  [unwired: 9 in]
          n180 = Variant To Data(error in=w424, type=w416, Variant=w423) -> (data=w417:cluster{string[]}[], error out=w422:errorcluster)
          n181 = Equal?(x=w417, y=w416) -> (x = y?=w418:bool)
          n182 = call <vilib>:"Error Cluster From Error Code.vi"("is warning? (False)"=w418, "error in (no error)"=w422, "error message (\"\")"="return mismatch" ("error message (\"\")"), "error code (0)"=5000) -> ("error out"=w421:errorcluster)  [unwired: 5 in]
        }
        frame "Cluster Array LuaToLabVIEW Embedded String Array Jagged" {
          w431 = cluster{string[]}[] [{["a", "s", "d"]}, {[]}, {["z", "x", "c"]}]
          n183 = call "New Instance.vi"("error in"=w440) -> ("error out"=w441:errorcluster, "GLue out"=w442:refnum<class "class.GLue.lvclass">)  [unwired: 9 in]
          n184 = call "Execute Script.vi"("Script"="g = require 'glue'\nout = g.clusterArray()\nout[1] = g.cluster(g.stringArray('a','s','d'))\nout[2] = g.cluster(g.stringArray())\nout[3] = g.cluster(g.stringArray('z','x','c'))\nreturn out", "error in"=w441, "GLue in"=w442) -> ("error out"=w443:errorcluster, "Return Data"=w438:variant, "GLue out"=w444:refnum<class "class.GLue.lvclass">)  [unwired: 6 in]
          n185 = call "Close Instance.vi"("error in"=w443, "GLue in"=w444) -> ("error out"=w439:errorcluster)  [unwired: 9 in]
          n186 = Variant To Data(error in=w439, type=w431, Variant=w438) -> (data=w432:cluster{string[]}[], error out=w437:errorcluster)
          n187 = Equal?(x=w432, y=w431) -> (x = y?=w433:bool)
          n188 = call <vilib>:"Error Cluster From Error Code.vi"("is warning? (False)"=w433, "error in (no error)"=w437, "error message (\"\")"="return mismatch" ("error message (\"\")"), "error code (0)"=5000) -> ("error out"=w436:errorcluster)  [unwired: 5 in]
        }
        frame "Cluster Array LuaToLabVIEW Embedded String Array Sparse" {
          w449 = 0 ("index")
          w450 = cluster{string[]}[] [{["a", "s", "d"]}, {[]}, {["z", "x", "c"]}]
          n189 = call "New Instance.vi"("error in"=w458) -> ("error out"=w459:errorcluster, "GLue out"=w460:refnum<class "class.GLue.lvclass">)  [unwired: 9 in]
          n190 = call "Execute Script.vi"("Script"="g = require 'glue'\nout = g.clusterArray()\nout[1] = g.cluster(g.stringArray('a','s','d'))\nout[2] = nil\nout[3] = g.cluster(g.stringArray('z','x','c'))\nreturn out", "error in"=w459, "GLue in"=w460) -> ("error out"=w461:errorcluster, "Return Data"=w456:variant, "GLue out"=w462:refnum<class "class.GLue.lvclass">)  [unwired: 6 in]
          n191 = call "Close Instance.vi"("error in"=w461, "GLue in"=w462) -> ("error out"=w457:errorcluster)  [unwired: 9 in]
          n192 = Variant To Data(error in=w457, type=w450, Variant=w456) -> (data=w451:cluster{string[]}[], error out=w455:errorcluster)
          n193 = Index Array(array=w451, index=w449) -> (element=w448:cluster{string[]})
          n194 = Index Array(array=w450, index=w449) -> (element=w447:cluster{string[]})
          n195 = Equal?(x=w448, y=w447) -> (x = y?=w446:bool)
          n196 = call <vilib>:"Error Cluster From Error Code.vi"("is warning? (False)"=w446, "error in (no error)"=w455, "error message (\"\")"="return mismatch" ("error message (\"\")"), "error code (0)"=5000) -> ("error out"=w454:errorcluster)  [unwired: 5 in]
        }
        frame "Cluster Array LuaToLabVIEW Multi Type" {
          n197 = call "New Instance.vi"("error in"=w469) -> ("error out"=w470:errorcluster, "GLue out"=w471:refnum<class "class.GLue.lvclass">)  [unwired: 9 in]
          n198 = call "Execute Script.vi"("Script"="g = require 'glue'\nout = g.clusterArray()\nout[1] = g.cluster(g.stringArray('a','s','d'))\nout[2] = g.cluster(true)\nout[3] = true\nreturn out", "error in"=w470, "GLue in"=w471) -> ("error out"=w472:errorcluster, "GLue out"=w473:refnum<class "class.GLue.lvclass">)  [unwired: 6 in, 1 out]
          n199 = call "Close Instance.vi"("error in"=w472, "GLue in"=w473) -> ("error out"=w464:errorcluster)  [unwired: 9 in]
          n200 = Unbundle By Name(w464) -> ("code"=w468:i32)
          n201 = Equal?(x=w468, y=9762) -> (x = y?=w466:bool)
          n202 = case shown="True" w466 {
            tunnel: [w475 errorcluster {"status"=FALSE, "code"=0, "source"=""} ("error out")] -> w465
            tunnel: w464 -> [w475 _]
            frame False {
            }
            frame True {
            }
          }
        }
        frame "Nested Cluster Array With Cluster And 2d Array" {
          n203 = control-ref of="This VI"() -> (w479:refnum<vi>)
          n204 = Bundle By Name(cluster=cluster{"ref":refnum<vi>, string[][]} {"ref"=refnum, [["a", "s"], ["z", "x"]]}, "ref"=w479) -> (w478:cluster{"ref":refnum<vi>, string[][]})
          n205 = Build Array(w478) -> (w477:cluster{"ref":refnum<vi>, string[][]}[])
          n206 = Bundle By Name(cluster=T2 {"ref"=refnum, "df"=[["a", "s"], ["z", "x"]], "asd"=[{"ref"=refnum, "df"=[["a", "s"], ["z", "x"]]}]}, "asd"=w477) -> (w486:T2)
          n207 = Build Array(w486, w486, w486, w486) -> (w485:T10)
          n208 = call "New Instance.vi"("error in"=w496) -> ("error out"=w497:errorcluster, "GLue out"=w498:refnum<class "class.GLue.lvclass">)  [unwired: 9 in]
          n209 = Bundle By Name(cluster=T3 {"arr"=[]}, "arr"=w485) -> (w487:T3)
          n210 = call "Execute Script.vi"("Script"="arg = ...\nreturn arg.arr[3].asd[1].ref", "error in"=w497, "Argument Data"=w487, "GLue in"=w498) -> ("error out"=w499:errorcluster, "Return Data"=w494:variant, "GLue out"=w500:refnum<class "class.GLue.lvclass">)  [unwired: 5 in]
          n211 = call "Close Instance.vi"("error in"=w499, "GLue in"=w500) -> ("error out"=w495:errorcluster)  [unwired: 9 in]
          n212 = Variant To Data(error in=w495, type=refnum<vi> refnum ("ref"), Variant=w494) -> (data=w482:refnum<vi>, error out=w493:errorcluster)
          n213 = control-ref of="This VI"() -> (w483:refnum<vi>)
          n214 = Equal?(x=w483, y=w482) -> (x = y?=w481:bool)
          n215 = call <vilib>:"Error Cluster From Error Code.vi"("is warning? (False)"=w481, "error in (no error)"=w493, "error message (\"\")"="return mismatch" ("error message (\"\")"), "error code (0)"=5000) -> ("error out"=w492:errorcluster)  [unwired: 5 in]
        }
        frame "Complex Cluster" {
          w502 = T11 {"a"=refnum, "z"=[{"array"=[["a", "s"], ["z", "x"]], "glue"=refnum, "q"={"a"=refnum, "z"=[{"array"=[["a", "s"], ["z", "x"]], "glue"=refnum}, {"array"=[["b", "c"], ["d", "e"]], "glue"=refnum}], "b"=[FALSE, TRUE, FALSE], "c"=refnum, "w"=[[1.0, 0.0, 0.0], [0.0, 0.0, 3.0]], "d"={"h"={"i"=bytes[0], "j"=variant, "g"=path ""}, {"t0"=timestamp(0 s since 1904-01-01), "dt"=1.0, "Y"=[]}}}}, {"array"=[["b", "c"], ["d", "e"]], "glue"=refnum, "q"={"a"=refnum, "z"=[{"array"=[["a", "s"], ["z", "x"]], "glue"=refnum}, {"array"=[["b", "c"], ["d", "e"]], "glue"=refnum}], "b"=[FALSE, TRUE, FALSE], "c"=refnum, "w"=[[1.0, 0.0, 0.0], [0.0, 0.0, 3.0]], "d"={"h"={"i"=bytes[0], "j"=variant, "g"=path ""}, {"t0"=timestamp(0 s since 1904-01-01), "dt"=1.0, "Y"=[]}}}}], "b"=[FALSE, TRUE, FALSE], "c"=refnum, "k 2"={"t0"=timestamp(0 s since 1904-01-01), "dt"=1.0, "Y"=[]}, "d"={"g"=path "", "h"={"i"=bytes[0], "j"=variant}}}  # asd
          n216 = call "New Instance.vi"("error in"=w510) -> ("error out"=w511:errorcluster, "GLue out"=w512:refnum<class "class.GLue.lvclass">)  [unwired: 9 in]
          n217 = call "Execute Script.vi"("Script"="arg = ...\nreturn arg", "error in"=w511, "Argument Data"=w502, "GLue in"=w512) -> ("error out"=w513:errorcluster, "Return Data"=w503:variant, "GLue out"=w514:refnum<class "class.GLue.lvclass">)  [unwired: 5 in]
          n218 = call "Close Instance.vi"("error in"=w513, "GLue in"=w514) -> ("error out"=w505:errorcluster)  [unwired: 9 in]
          n219 = Variant To Data(error in=w505, type=w502, Variant=w503) -> (error out=w504:errorcluster)  [unwired: 1 out]
          n220 = call <vilib>:"Error Cluster From Error Code.vi"("is warning? (False)"=TRUE, "error in (no error)"=w504, "error message (\"\")"="return mismatch" ("error message (\"\")"), "error code (0)"=5000) -> ("error out"=w509:errorcluster)  [unwired: 5 in]
        }
        frame "Basic Nested Cluster" {
          w519 = T4 {"a"={"bool"=TRUE, "number"=0, "string"=""}, "b"={"bool"=TRUE, "number"=0, "string"="", "c"={"bool"=TRUE, "number"=0, "string"=""}}}
          n221 = call "New Instance.vi"("error in"=w526) -> ("error out"=w527:errorcluster, "GLue out"=w528:refnum<class "class.GLue.lvclass">)  [unwired: 9 in]
          n222 = call "Execute Script.vi"("Script"="arg = ...\narg.a.bool = false\narg.a.number = 1\narg.a.string = 'a'\narg.b.bool = false\narg.b.number = 2\narg.b.string = 'b'\narg.b.c.bool = true\narg.b.c.number = 3\narg.b.c.string = 'c'\nreturn arg", "error in"=w527, "Argument Data"=w519, "GLue in"=w528) -> ("error out"=w529:errorcluster, "Return Data"=w524:variant, "GLue out"=w530:refnum<class "class.GLue.lvclass">)  [unwired: 5 in]
          n223 = call "Close Instance.vi"("error in"=w529, "GLue in"=w530) -> ("error out"=w525:errorcluster)  [unwired: 9 in]
          n224 = Variant To Data(error in=w525, type=w519, Variant=w524) -> (data=w517:T4, error out=w523:errorcluster)
          n225 = Equal?(x=w517, y=T4 {"a"={"bool"=FALSE, "number"=1, "string"="a"}, "b"={"bool"=FALSE, "number"=2, "string"="b", "c"={"bool"=TRUE, "number"=3, "string"="c"}}}) -> (x = y?=w516:bool)
          n226 = call <vilib>:"Error Cluster From Error Code.vi"("is warning? (False)"=w516, "error in (no error)"=w523, "error message (\"\")"="return mismatch" ("error message (\"\")"), "error code (0)"=5000) -> ("error out"=w522:errorcluster)  [unwired: 5 in]
        }
        frame "Nested Cluster Within Variant" {
          w533 = T12 {"bool"=TRUE, "number"=0, "string"="", "c"={"bool"=TRUE, "number"=0, "string"=""}}  # b
          n227 = call "New Instance.vi"("error in"=w541) -> ("error out"=w542:errorcluster, "GLue out"=w543:refnum<class "class.GLue.lvclass">)  [unwired: 9 in]
          n228 = Bundle By Name(cluster=T5 {"a"={"bool"=TRUE, "number"=0, "string"=""}, "data"=variant}, "data"=w533) -> (w537:T5)
          n229 = call "Execute Script.vi"("Script"="arg = ...\n\nreturn arg", "error in"=w542, "Argument Data"=w537, "GLue in"=w543) -> ("error out"=w544:errorcluster, "Return Data"=w539:variant, "GLue out"=w545:refnum<class "class.GLue.lvclass">)  [unwired: 5 in]
          n230 = call "Close Instance.vi"("error in"=w544, "GLue in"=w545) -> ("error out"=w540:errorcluster)  [unwired: 9 in]
          n231 = Variant To Data(error in=w540, type=w537, Variant=w539) -> (data=w535:T5, error out=w536:errorcluster)
          n232 = Unbundle By Name(w535) -> ("data"=w534:variant)
          n233 = Variant To Data(error in=w536, type=w533, Variant=w534) -> (error out=w532:errorcluster)  [unwired: 1 out]
        }
        frame "Nested Cluster With Arrays" {
          w548 = T6 {"a"={"numbers"=[1, 2, 3], "bools"=[FALSE, FALSE, FALSE], "strings"=["a", "b", "c"]}, "b"={"numbers"=[1, 2, 3], "bools"=[FALSE, FALSE, FALSE], "strings"=["a", "b", "c"], "c"={"numbers"=[1, 2, 3], "bools"=[FALSE, FALSE, FALSE], "strings"=["a", "b", "c"]}}}
          n234 = call "New Instance.vi"("error in"=w557) -> ("error out"=w558:errorcluster, "GLue out"=w559:refnum<class "class.GLue.lvclass">)  [unwired: 9 in]
          n235 = call "Execute Script.vi"("Script"="arg = ...\narg.b.c.bools[2] = true\narg.b.numbers[2] = 5\narg.a.strings[2] = 'd'\nreturn arg", "error in"=w558, "Argument Data"=w548, "GLue in"=w559) -> ("error out"=w560:errorcluster, "Return Data"=w555:variant, "GLue out"=w561:refnum<class "class.GLue.lvclass">)  [unwired: 5 in]
          n236 = call "Close Instance.vi"("error in"=w560, "GLue in"=w561) -> ("error out"=w556:errorcluster)  [unwired: 9 in]
          n237 = Variant To Data(error in=w556, type=w548, Variant=w555) -> (data=w550:T6, error out=w554:errorcluster)
          n238 = Equal?(x=w550, y=T6 {"a"={"numbers"=[1, 2, 3], "bools"=[FALSE, FALSE, FALSE], "strings"=["a", "d", "c"]}, "b"={"numbers"=[1, 5, 3], "bools"=[FALSE, FALSE, FALSE], "strings"=["a", "b", "c"], "c"={"numbers"=[1, 2, 3], "bools"=[FALSE, TRUE, FALSE], "strings"=["a", "b", "c"]}}}) -> (x = y?=w549:bool)
          n239 = call <vilib>:"Error Cluster From Error Code.vi"("is warning? (False)"=w549, "error in (no error)"=w554, "error message (\"\")"="return mismatch" ("error message (\"\")"), "error code (0)"=5000) -> ("error out"=w553:errorcluster)  [unwired: 5 in]
        }
        frame "Nested Cluster from lua" {
          w563 = T13 {"clus2"={"clus1"={TRUE, 5, "string"="asd"}, "sdf"}, 1, "string"="dfg"}  # clus3
          n240 = call "New Instance.vi"("error in"=w572) -> ("error out"=w573:errorcluster, "GLue out"=w574:refnum<class "class.GLue.lvclass">)  [unwired: 9 in]
          n241 = call "Execute Script.vi"("Script"="glue = require 'glue'\n\nclus1 = glue.cluster(true,5,'asd')\nclus2 = glue.cluster(clus1,'sdf')\nclus3 = glue.cluster(clus2,1,'dfg')\n\nreturn clus3", "error in"=w573, "GLue in"=w574) -> ("error out"=w575:errorcluster, "Return Data"=w570:variant, "GLue out"=w576:refnum<class "class.GLue.lvclass">)  [unwired: 6 in]
          n242 = call "Close Instance.vi"("error in"=w575, "GLue in"=w576) -> ("error out"=w571:errorcluster)  [unwired: 9 in]
          n243 = Variant To Data(error in=w571, type=w563, Variant=w570) -> (data=w565:T13, error out=w569:errorcluster)
          n244 = Equal?(x=w565, y=w563) -> (x = y?=w564:bool)
          n245 = call <vilib>:"Error Cluster From Error Code.vi"("is warning? (False)"=w564, "error in (no error)"=w569, "error message (\"\")"="return mismatch" ("error message (\"\")"), "error code (0)"=5000) -> ("error out"=w568:errorcluster)  [unwired: 5 in]
        }
        frame "Circular Cluster Reference From Lua" {
          n246 = call "New Instance.vi"("error in"=w580) -> ("error out"=w581:errorcluster, "GLue out"=w582:refnum<class "class.GLue.lvclass">)  [unwired: 9 in]
          n247 = call "Execute Script.vi"("Script"="glue = require 'glue'\n\nclus1 = glue.cluster(true)\nclus2 = glue.cluster(true)\nclus2.ref = clus1\nclus1.ref = clus2\n\nreturn clus1", "error in"=w581, "GLue in"=w582) -> ("error out"=w583:errorcluster, "GLue out"=w584:refnum<class "class.GLue.lvclass">)  [unwired: 6 in, 1 out]
          n248 = call "Close Instance.vi"("error in"=w583, "GLue in"=w584) -> ("error out"=w579:errorcluster)  [unwired: 9 in]
          n249 = case shown="Error" w579 {
            selector: w579 -> [_ w590]
            tunnel: [errorcluster {"status"=TRUE, "code"=5000, "source"="exception expected"} ("error IO") w591] -> w578
            frame No Error {
            }
            frame Error {
              n250 = Unbundle By Name(w590) -> ("code"=w587:i32)
              n251 = Equal?(x=w587, y=9758) -> (x = y?=w588:bool)
              n252 = call <vilib>:"Error Cluster From Error Code.vi"("is warning? (False)"=w588, "error message (\"\")"="wrong error generated" ("error message (\"\")"), "error code (0)"=w587) -> ("error out"=w591:errorcluster)  [unwired: 6 in]
            }
          }
        }
      }
    }
    frame Error {
    }
  }
  "Return Data" <- w1
  "error out" <- w2
